vi "Button State Get.vi"(8 "error in (no error)":errorcluster) -> (0 "error out":errorcluster, 2 "Button State":bool)   [LabVIEW 2023, in "Haptic Prog Interface.lvlib"]
doc: "Returns the button state of the haptic pen.\n\n<b>Button State:</b> Returns the boolean state of the pen button."
uses:
  Haptic Prog Interface.lvlib
  src/x64/Debug/Haptic Programming Interface.dll
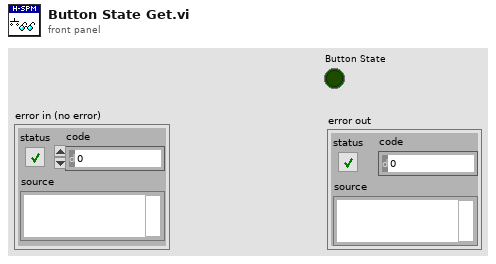
[diagram p1: front panel]
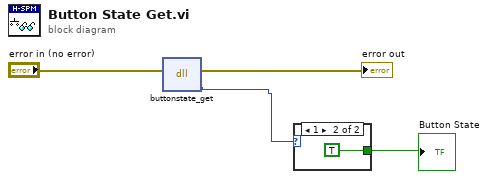
[diagram p0: block diagram]
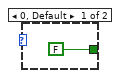
[diagram p2: hidden frame]
diagram:
  n1 = dll-call lib="C:/Users/cjwel/Documents/GitHub/Haptic-Programming-Interface/src/x64/Debug/Haptic Programming Interface.dll" fn="buttonstate_get"(error in="error in (no error)") -> (error out=→"error out":errorcluster, "state"=w1:i8)  [unwired: 4 in, 1 out]
  n2 = case shown="1" w1 {
    tunnel: [FALSE TRUE] -> w2
    frame 0, Default {
    }
    frame 1 {
    }
  }
  "Button State" <- w2
